vi "PS_ManCMD.vi"(2 "Power Sup: T-On/F-Off":bool, 3 "error in":errorcluster, 4 "Command":string, 5 "VISA resource name":refnum<visa-resource-name>="COM3") -> (0 "error out":errorcluster)   [LabVIEW 2017]
panel:
  # "This command is for\nAgilent E3631A Triple Output DC Power Supply\n\nCommunication port: RS-232, 9600 Baud, None Parity,  8 Bits\n\nThis SubVI enables manually enter values to power supply"
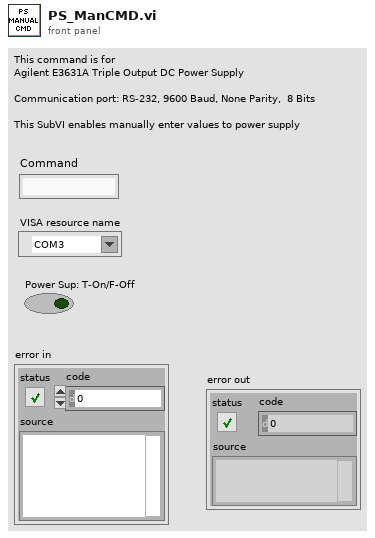
[diagram p1: front panel]
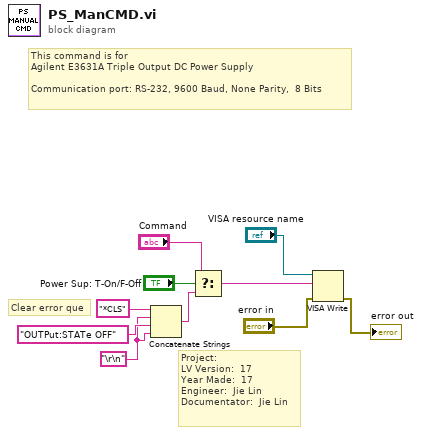
[diagram p0: block diagram]
diagram:
  w8 = "\r\n"
  # "Project:  \nLV Version:  17\nYear Made:  17\nEngineer:  Jie Lin\nDocumentator:  Jie Lin"
  # "Clear error que"
  # "This command is for\nAgilent E3631A Triple Output DC Power Supply\n\nCommunication port: RS-232, 9600 Baud, None Parity,  8 Bits"
  n1 = Concatenate Strings("*CLS" ("write buffer"), w8, "OUTPut:STATe OFF" ("write buffer"), w8) -> (w6:string)
  n2 = Select(t="Command", s="Power Sup: T-On/F-Off", f=w6) -> (s? t:f=w5:string)
  n3 = VISA Write(VISA resource name="VISA resource name", write buffer=w5, error in (no error)="error in") -> (error out=→"error out":errorcluster)  [unwired: 2 out]
